vi "Settings Dialog.vi"(8 "error in (no error)":errorcluster, 9 "UI State":T1, 10 "Message Queues":T2, 11 "PRM State Cluster In":T6={"PRM Config"={"GUID"="", "Drop Coords"={"Horizontal"=0, "Vertical"=0}, "Process Name"="", "User name"="", "Queue Name"="", "Settings"={"Cycle Period"=500.0, "PID 2 Parameters"={"Input Device"=enum."Default", "Output Device"=enum."Default", "Setpoint"=0.0, "PID gains"={"proportional gain (Kc)"=1.0, "integral time (Ti, min)"=0.01, "derivative time (Td, min)"=0.0}, "output range"={"output low"=0.0, "output high"=100.0}}, "Manual Entry"=0.0, "Auto?"=TRUE, "4-20mA Input Settings"={"Input Channel "=0}, "4-20mA Out Settings"={"Output DAQ Task"=""}, "Input Channel Tag Name "=""}, "Settings Load Count"=0}, "State"=enum."Idle", "Start Time"=timestamp(0 s since 1904-01-01), "Current Time"=timestamp(0 s since 1904-01-01), "First Iteration"=FALSE, "Data"={"4-20mA Input"=0.0, "PID 2 Process Variable"=0.0, "PID 2 Output"=0.0, "4-20mA Output"=0.0}} {"PRM Config"."Settings"."PID 2 Parameters"."output range"."output low" format="%.2f"; "PRM Config"."Settings"."PID 2 Parameters"."output range"."output high" min=0.0 max=100.0 format="%.2f"; "PRM Config"."Settings"."PID 2 Parameters"."PID gains"."derivative time (Td, min)" format="%.3f"; "PRM Config"."Settings"."PID 2 Parameters"."PID gains"."integral time (Ti, min)" format="%.3f"; "PRM Config"."Settings"."PID 2 Parameters"."PID gains"."proportional gain (Kc)" format="%.3f"}) -> (0 "error out":errorcluster, 1 "Cancelled?":bool=TRUE, 2 "UI Refresh Needed?":bool, 3 "PRM State Cluster Out":T6={"PRM Config"={"GUID"="", "Drop Coords"={"Horizontal"=0, "Vertical"=0}, "Process Name"="", "User name"="", "Queue Name"="", "Settings"={"Cycle Period"=500.0, "PID 2 Parameters"={"Input Device"=enum."Default", "Output Device"=enum."Default", "Setpoint"=0.0, "PID gains"={"proportional gain (Kc)"=1.0, "integral time (Ti, min)"=0.01, "derivative time (Td, min)"=0.0}, "output range"={"output low"=0.0, "output high"=100.0}}, "Manual Entry"=0.0, "Auto?"=TRUE, "4-20mA Input Settings"={"Input Channel "=0}, "4-20mA Out Settings"={"Output DAQ Task"=""}, "Input Channel Tag Name "=""}, "Settings Load Count"=0}, "State"=enum."Idle", "Start Time"=timestamp(0 s since 1904-01-01), "Current Time"=timestamp(0 s since 1904-01-01), "First Iteration"=FALSE, "Data"={"4-20mA Input"=0.0, "PID 2 Process Variable"=0.0, "PID 2 Output"=0.0, "4-20mA Output"=0.0}} {"PRM Config"."Settings"."PID 2 Parameters"."output range"."output low" format="%.2f"; "PRM Config"."Settings"."PID 2 Parameters"."output range"."output high" min=0.0 max=100.0 format="%.2f"; "PRM Config"."Settings"."PID 2 Parameters"."PID gains"."derivative time (Td, min)" format="%.3f"; "PRM Config"."Settings"."PID 2 Parameters"."PID gains"."integral time (Ti, min)" format="%.3f"; "PRM Config"."Settings"."PID 2 Parameters"."PID gains"."proportional gain (Kc)" format="%.3f"})   [LabVIEW 2018, in "4-20mA Module.lvlib"]
uses:
  4-20mA Module.lvlib
  Controls/4-20mA Module State Cluster.ctl
  Controls/4-20mA Module Config Cluster.ctl
  <vilib>/Utility/miscctls.llb/LVPoint32TypeDef.ctl
  Controls/4-20mA Module Settings Cluster.ctl
  Pressure Transmitter/Pressure Transmitter Device Settings.ctl
  Pressure Reg Module/Pressure Regulator Device Settings.ctl
  Measure Instrument/State Enum.ctl
  Controls/4-20mA Message Queues.ctl
  support/Message Queue/Message Cluster.ctl
  controls/UI State.ctl
  Tag VIs/Tag FGV Operation Enum.ctl
  <vilib>/Utility/miscctls.llb/LVMinMaxIncTypeDef.ctl
  support/Message Queue/Enqueue Message (Single).vi
  Settings/Settings.lvlib
  Pressure Transmitter/Pressure Transmitter Library.lvlib
  Shared Variables/Dynamic Shared Variables.lvlib
  Pressure Reg Module/Pressure Regulator Library.lvlib
  support/Support Library.lvlib
  support/Message Queue/Message Queue.lvlib
  Flow Regulator/Pressure Reg Module/Flow Regulator Library.lvlib
  <vilib>/Utility/xml.llb/Write to XML File(string).vi
  Measure Instrument/Feed Module Engine.lvlib
panel:
  in  "Module Name":string
  in  "Start":bool
  in  "Stop":bool
  in  "Pressure Regulator Configuration":T5={"Cycle Period"=500.0, "PID 2 Parameters"={"Input Device"=enum."Default", "Output Device"=enum."Default", "Setpoint PSIA"=0.0, "PID gains"={"proportional gain (Kc)"=1.0, "integral time (Ti, min)"=0.01, "derivative time (Td, min)"=0.0}, "output range"={"output low"=0.0, "output high"=100.0}}, "Manual PSIA"=0.0, "Auto?"=TRUE, "4-20mA Input Settings"={"Input Channel "=0}, "Out Settings"={"Output DAQ Task"=""}, "Simulated"=FALSE} {"4-20mA Input Settings"."Input Channel" items=["Default", "TT0", "PT0", "PR 1:4-20mA Input", "PR 1:PID2Out", "PR 1:4-20mA Output", "PR 1:Input Device Disconnected", "PR 1:Output Device Disconnected"]; "Manual PSIA" min=0.0 max=50.0; "PID 2 Parameters"."output range"."output low" format="%.2f"; "PID 2 Parameters"."output range"."output high" min=0.0 max=100.0 format="%.2f"; "PID 2 Parameters"."PID gains"."derivative time (Td, min)" format="%.3f"; "PID 2 Parameters"."PID gains"."integral time (Ti, min)" format="%.3f"; "PID 2 Parameters"."PID gains"."proportional gain (Kc)" format="%.3f"}
  in  "Cancel Button":bool
  in  "OK Button":bool
  # "Output Settings"
  # "Input Settings"
  # "Instrument Settings"
  # "Instrument Settings"
  # "Instrument Settings"
  # "Instrument Settings"
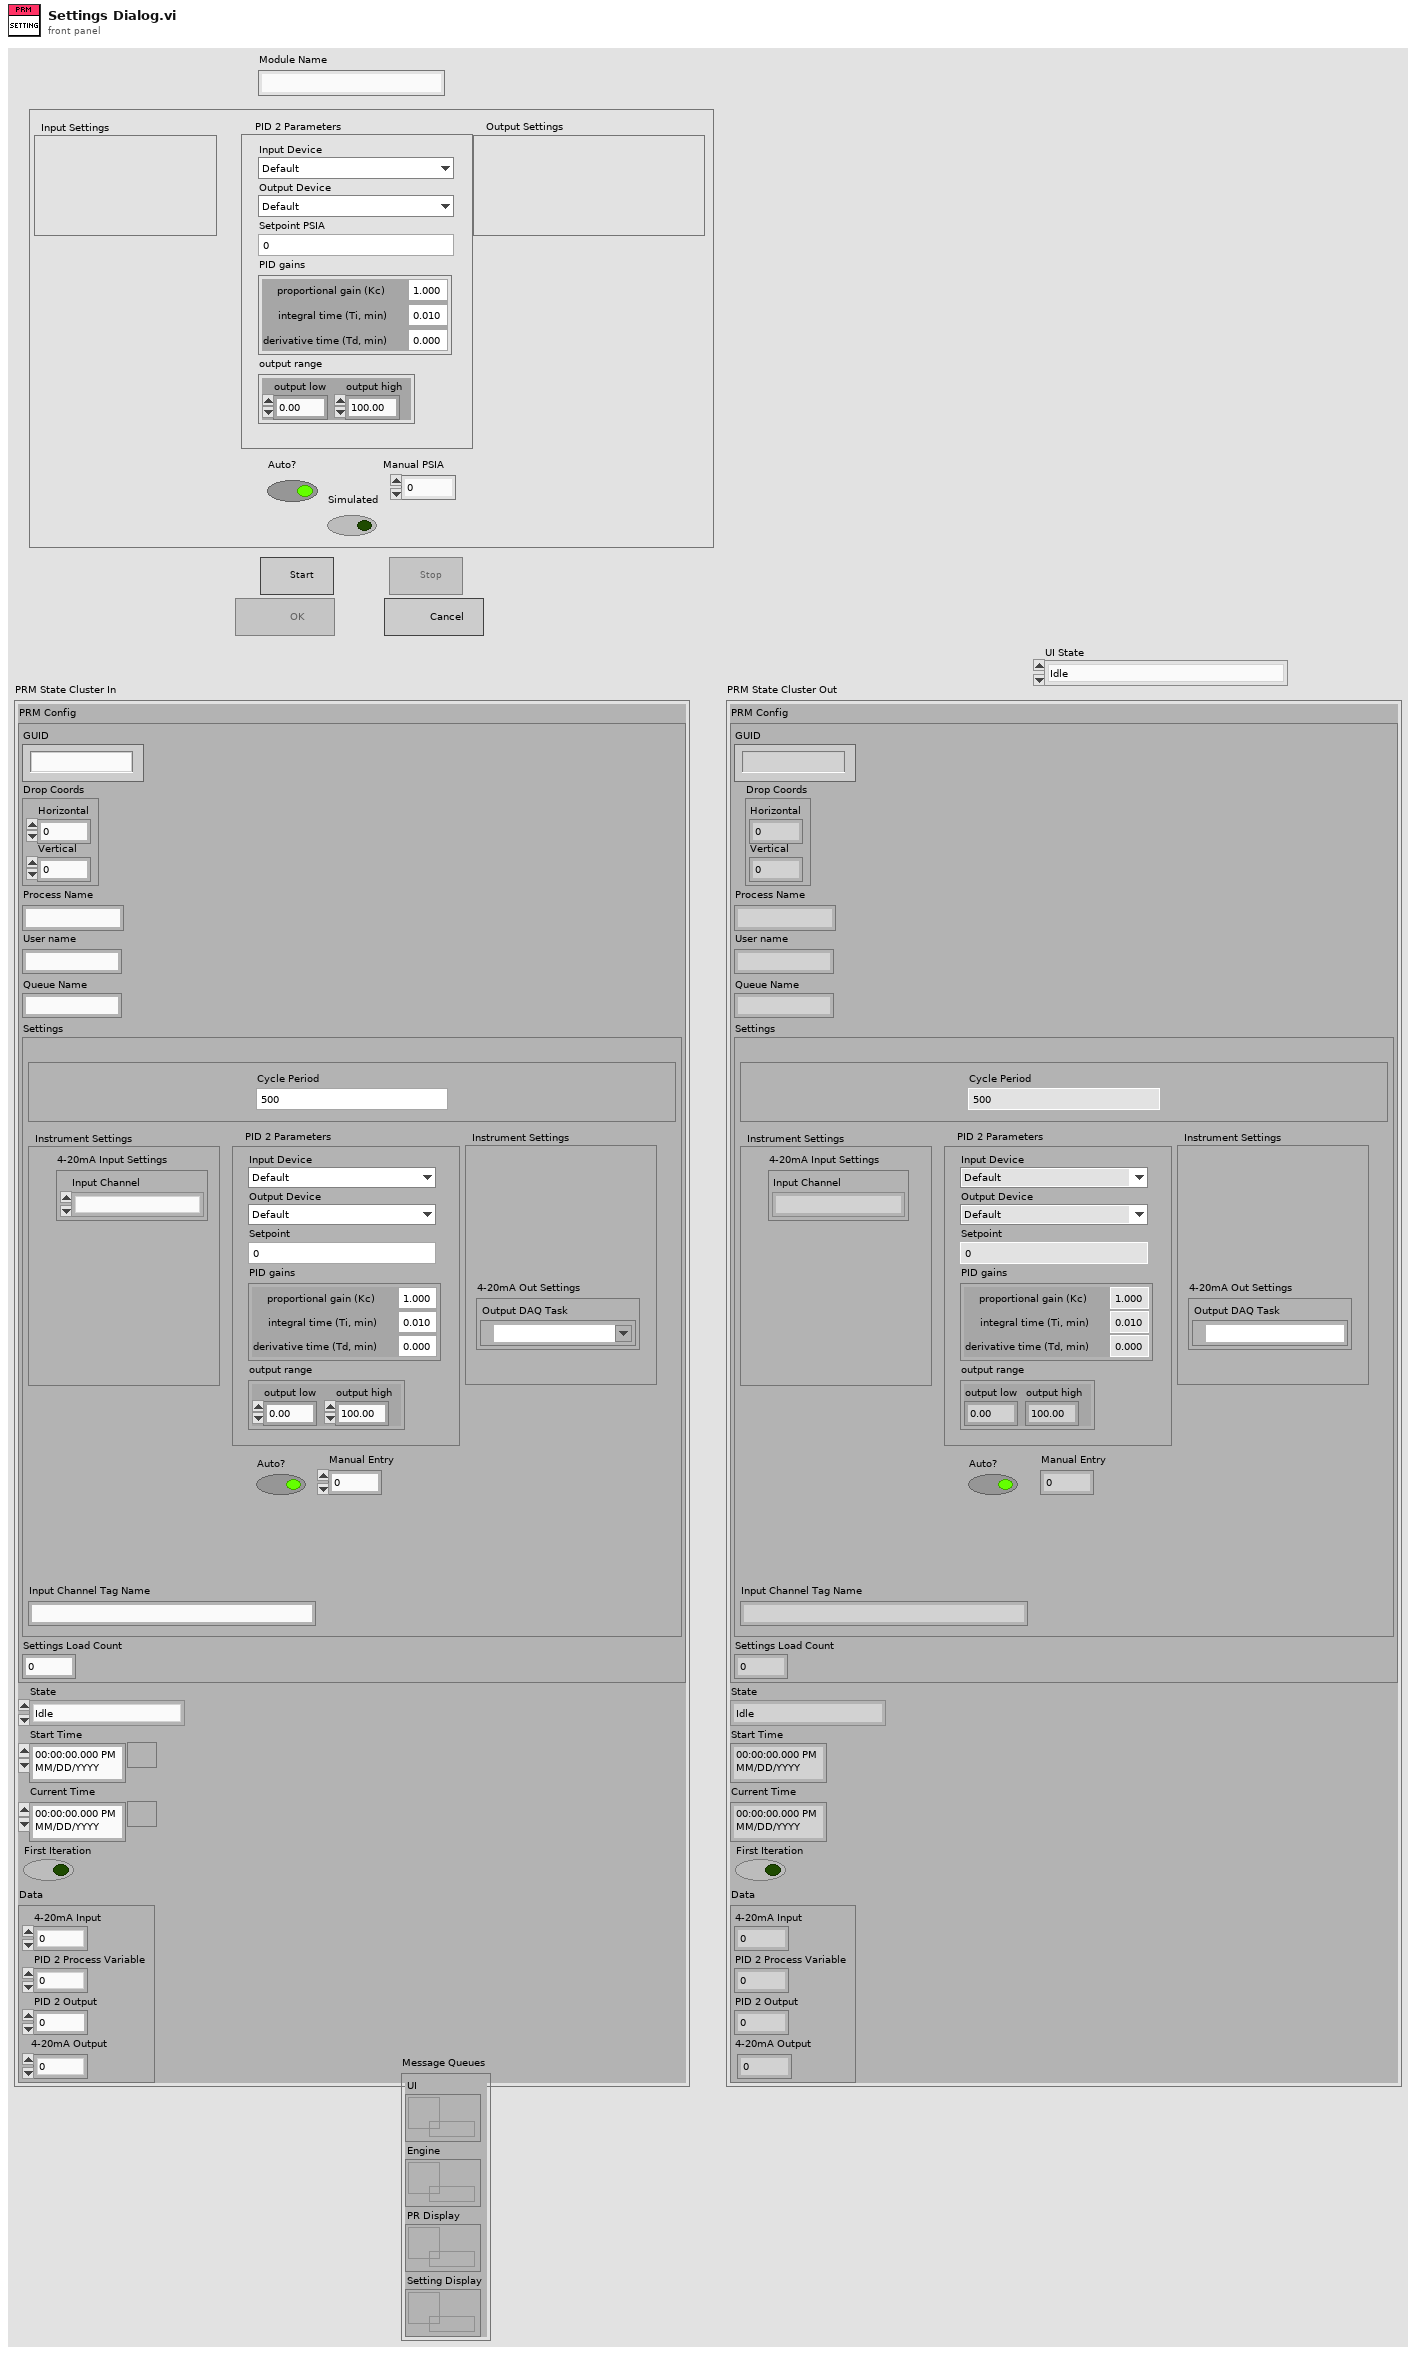
[diagram p1: front panel]
types:
  T1 = typedef "UI State.ctl" = enum16{"Idle", "Acquiring and Logging", "Waiting for Exit", "Waiting for Exit (Acq Stopped)", "Waiting for Exit (Log Stopped)", "Waiting for Stop", "Waiting for Stop (Acq Stopped)", "Waiting for Stop (Log Stopped)"}
  T2 = typedef "4-20mA Module.lvlib/4-20mA Message Queues.ctl" = cluster{"UI":refnum<queue>, "Engine":refnum<queue>, "PR Display":refnum<queue>, "Setting Display":refnum<queue>}
  T3 = typedef "Pressure Transmitter Library.lvlib/Pressure Transmitter Device Settings.ctl" = cluster{"Input Channel ":u16}
  T4 = typedef "Pressure Regulator Library.lvlib/Pressure Regulator Device Settings.ctl" = cluster{"Output DAQ Task":refnum<k21>}
  T5 = cluster{"Cycle Period":dbl, "PID 2 Parameters":cluster{"Input Device":enum16{"Default", "4-20mA"}, "Output Device":enum16{"Default", "Equilibar Pressure Reg", "Flow Regulator"}, "Setpoint PSIA":dbl, "PID gains":cluster{"proportional gain (Kc)":dbl, "integral time (Ti, min)":dbl, "derivative time (Td, min)":dbl}, "output range":cluster{"output low":dbl, "output high":dbl}}, "Manual PSIA":dbl, "Auto?":bool, "4-20mA Input Settings":T3, "Out Settings":T4, "Simulated":bool}
  T6 = typedef "4-20mA Module.lvlib/4-20mA Module State Cluster.ctl" = cluster{"PRM Config":T7, "State":T10, "Start Time":timestamp, "Current Time":timestamp, "First Iteration":bool, "Data":cluster{"4-20mA Input":dbl, "PID 2 Process Variable":dbl, "PID 2 Output":dbl, "4-20mA Output":dbl}}
  T7 = typedef "4-20mA Module.lvlib/4-20mA Module Config Cluster.ctl" = cluster{"GUID":string, "Drop Coords":T8, "Process Name":string, "User name":string, "Queue Name":string, "Settings":T9, "Settings Load Count":i32}
  T8 = typedef "LVPoint32TypeDef.ctl" = cluster{"Horizontal":i32, "Vertical":i32}
  T9 = typedef "4-20mA Module.lvlib/4-20mA Module Settings Cluster.ctl" = cluster{"Cycle Period":dbl, "PID 2 Parameters":cluster{"Input Device":enum16{"Default", "4-20mA"}, "Output Device":enum16{"Default", "Equilibar Pressure Reg", "Flow Regulator"}, "Setpoint":dbl, "PID gains":cluster{"proportional gain (Kc)":dbl, "integral time (Ti, min)":dbl, "derivative time (Td, min)":dbl}, "output range":cluster{"output low":dbl, "output high":dbl}}, "Manual Entry":dbl, "Auto?":bool, "4-20mA Input Settings":T3, "4-20mA Out Settings":T4, "Input Channel Tag Name ":string}
  T10 = typedef "Feed Module.lvlib/Feed Module Engine.lvlib/State Enum.ctl" = enum16{"Measuring", "Idle", "Paused"}
  T11 = typedef "Tag FGV Operation Enum.ctl" = enum16{"Init", "Set Notification Queue", "Create Tag", "Commit", "Write Tag (Numeric)", "Write Tag (Boolean)", "Read All Tags", "Read One Tag", "Delete Tag Category", "Set Alarm Parameters (Numeric)", "Set Alarm Parameters (Boolean)", "Enable All Alarms", "Disable All Alarms", "Delete All Tags", "Read Alarms", "Ack Alarm", "Read Alarm Parameters (Numeric)", "Read Alarm Parameters (Boolean)"}
  T12 = enum8{"Enabled", "Disabled", "Disabled and Grayed Out"}
  T13 = typedef "LVMinMaxIncTypeDef.ctl" = cluster{"Minimum":dbl, "Maximum":dbl, "Increment":dbl}
  T14 = cluster{"Input Device":enum16{"Default", "4-20mA"}, "Output Device":enum16{"Default", "Equilibar Pressure Reg", "Flow Regulator"}, "Setpoint":dbl, "PID gains":cluster{"proportional gain (Kc)":dbl, "integral time (Ti, min)":dbl, "derivative time (Td, min)":dbl}, "output range":cluster{"output low":dbl, "output high":dbl}}
  T15 = cluster{"Input Device":enum16{"Default", "4-20mA"}, "Output Device":enum16{"Default", "Equilibar Pressure Reg", "Flow Regulator"}, "Setpoint PSIA":dbl, "PID gains":cluster{"proportional gain (Kc)":dbl, "integral time (Ti, min)":dbl, "derivative time (Td, min)":dbl}, "output range":cluster{"output low":dbl, "output high":dbl}}
  T16 = enum16{"Default", "Equilibar Pressure Reg", "Flow Regulator"}
  T17 = cluster{"Numeric Text.Text":dbl, "Numeric Text.Text":dbl, "Numeric Text.Text":dbl}
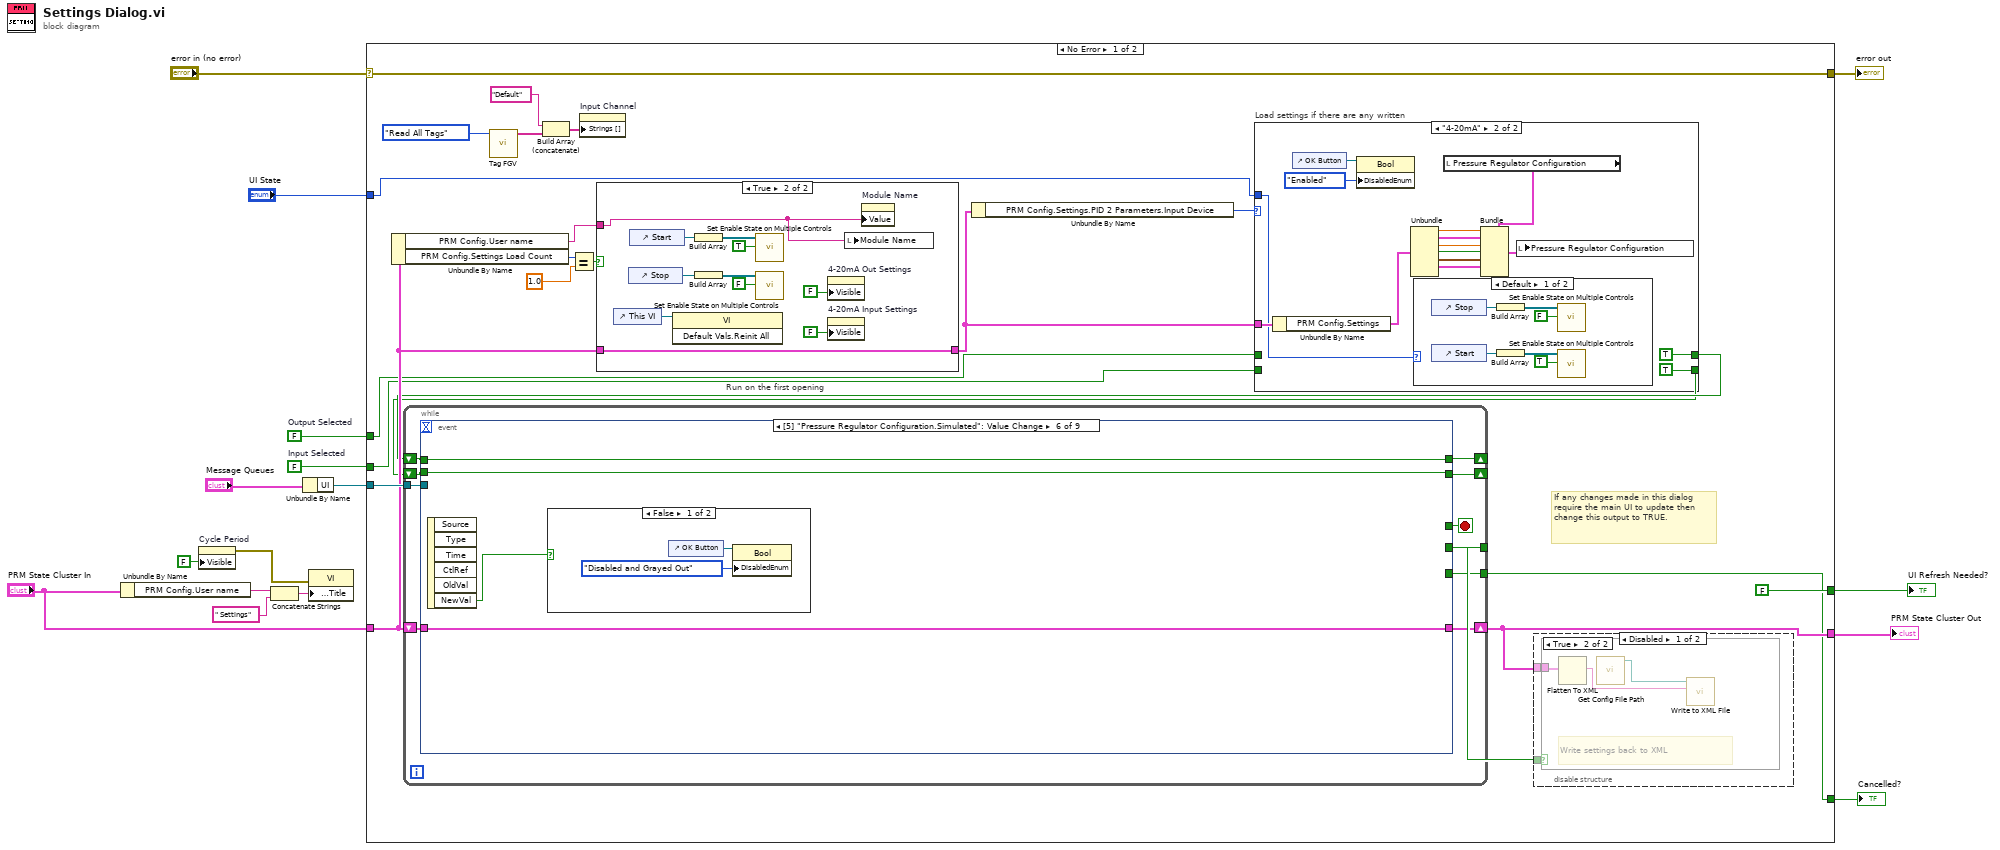
[diagram p0: block diagram]
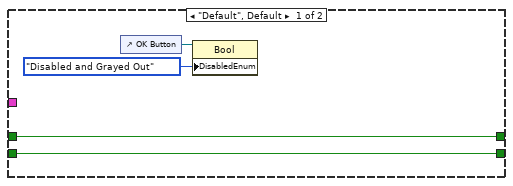
[diagram p4: hidden frame]
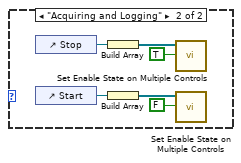
[diagram p5: hidden frame]
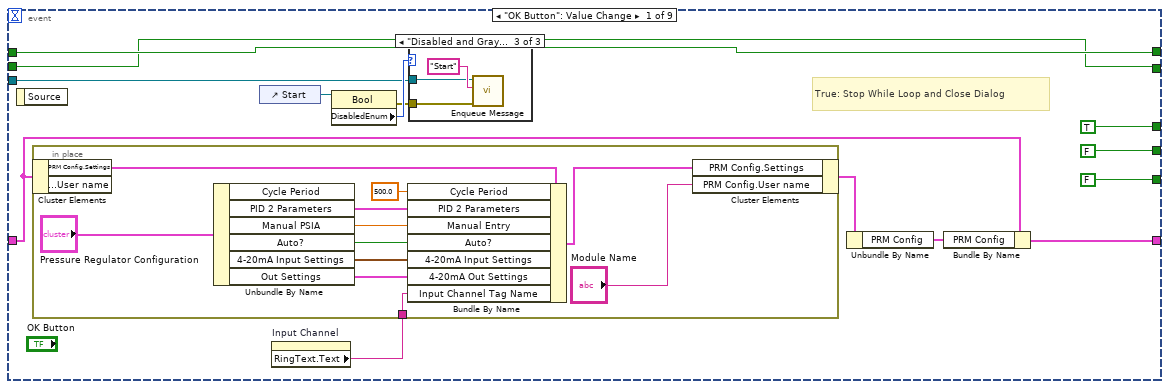
[diagram p7: hidden frame]
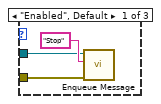
[diagram p8: hidden frame]
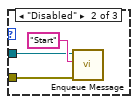
[diagram p9: hidden frame]
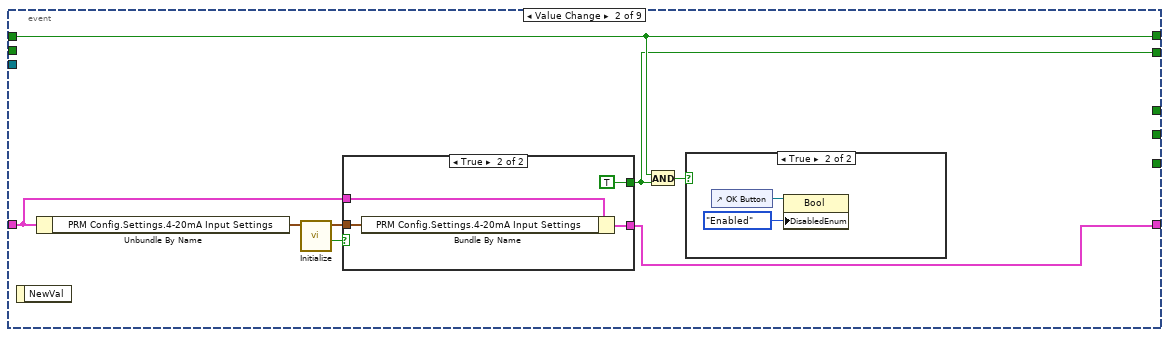
[diagram p10: hidden frame]
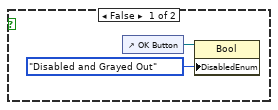
[diagram p11: hidden frame]
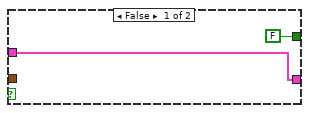
[diagram p12: hidden frame]
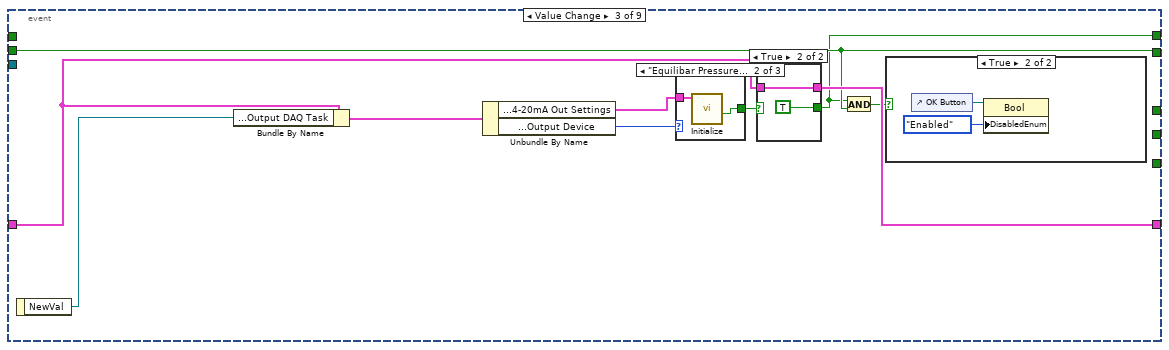
[diagram p13: hidden frame]
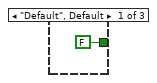
[diagram p14: hidden frame]
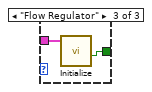
[diagram p15: hidden frame]
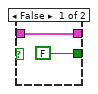
[diagram p16: hidden frame]
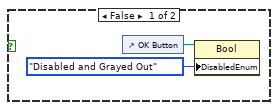
[diagram p17: hidden frame]
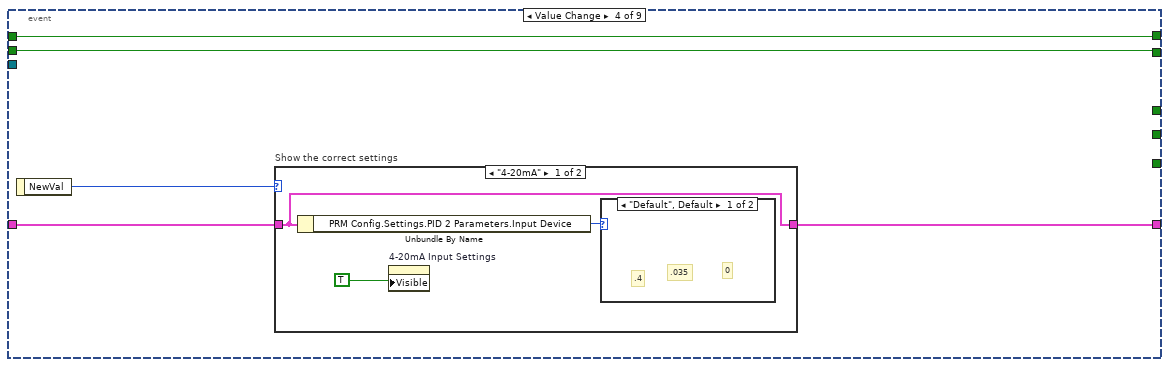
[diagram p18: hidden frame]
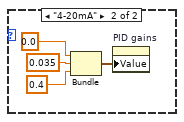
[diagram p19: hidden frame]
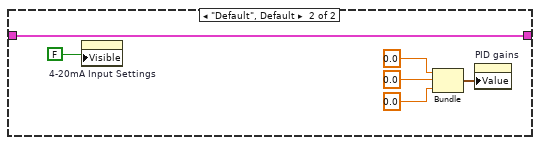
[diagram p20: hidden frame]
diagram:
  w5 = FALSE  # Input Selected
  w6 = FALSE  # Output Selected
  n1 = Unbundle By Name("PRM State Cluster In") -> ("PRM Config.User name"=w13:string)
  n2 = property on="Cycle Period" class="DigNum (strict)"("Visible"=FALSE) -> (error out=w1:errorcluster)  [unwired: 2 in, 1 out]
  n3 = Concatenate Strings(w13, " Settings" ("string")) -> (w12:string)
  n4 = Unbundle By Name("Message Queues") -> ("UI"=w7:refnum<queue>)
  n5 = property class="VI"(error in=w1, "Front Panel.Title"=w12) -> ()  [unwired: 1 in, 2 out]
  n6 = case shown="No Error" "error in (no error)" {
    selector: "error in (no error)" -> [w38 w237]
    tunnel: [w38 w237] -> w16
    tunnel: "PRM State Cluster In" -> [w25 w236]
    tunnel: [w36 w236] -> w10
    tunnel: [FALSE ("UI Refresh Needed?") _] -> w15
    tunnel: [w35 TRUE ("UI Refresh Needed?")] -> w14
    tunnel: w7 -> [w26 _]
    tunnel: w6 -> [w24 _]
    tunnel: w5 -> [w23 _]
    tunnel: "UI State" -> [w20 _]
    frame No Error {
      # "If any changes made in this dialog require the main UI to update then change this output to TRUE."
      n7 = Unbundle By Name(w25) -> ("PRM Config.User name"=w19:string, "PRM Config.Settings Load Count"=w34:i32)
      n8 = call "Tag FGV.vi"("Operation"=Tag_FGV_Operation_Enum."Read All Tags") -> ("Tag Names"=w18:string[])  [unwired: 7 in, 7 out]
      n9 = Build Array (concatenate)("Default", w18) -> (w27:string[])
      n10 = Equal?(x=w34, y=1.0) -> (x = y?=w31:bool)
      n11 = property on="Input Channel" class="Ring (strict)"("Strings []"=w27) -> ()  [unwired: 2 in, 2 out]
      n12 = case "Run on the first opening" shown="True" w31 {
        tunnel: w25 -> [w75 w85]
        tunnel: [w75 w85] -> w29
        tunnel: w19 -> [_ w76]
        frame False {
        }
        frame True {
          n13 = control-ref of="This VI"() -> (w86:refnum<vi>)
          n14 = control-ref of="Stop"() -> (w81:refnum<vi>)
          n15 = control-ref of="Start"() -> (w82:refnum<vi>)
          n16 = invoke class="VI" method="Default Vals.Reinit All"(reference=w86) -> ()  [unwired: 2 in, 3 out]
          n17 = Build Array(w82) -> (w80:refnum<vi>[])
          n18 = Build Array(w81) -> (w79:refnum<vi>[])
          n19 = call "Set Enable State on Multiple Controls.vi"("Enable?"=TRUE, "Controls"=w80) -> ()  [unwired: 10 in]
          n20 = call "Set Enable State on Multiple Controls.vi"("Enable?"=FALSE, "Controls"=w79) -> ()  [unwired: 10 in]
          n21 = property on="4-20mA Out Settings" class="Clust (strict)"("Visible"=FALSE) -> ()  [unwired: 2 in, 2 out]
          n22 = property on="4-20mA Input Settings" class="Clust (strict)"("Visible"=FALSE) -> ()  [unwired: 2 in, 2 out]
          n23 = local write "Module Name"(w76) -> ()
          n24 = property on="Module Name" class="Str"("Value"=w76) -> ()  [unwired: 2 in, 2 out]
        }
      }
      n25 = Unbundle By Name(w29) -> ("PRM Config.Settings.PID 2 Parameters.Input Device"=w30:enum16{"Default", "4-20mA"})
      n26 = case "Load settings if there are any written" shown="\"4-20mA\"" w30 {
        tunnel: w29 -> [_ w56]
        tunnel: w24 -> [w45 _]
        tunnel: w23 -> [w44 _]
        tunnel: [w45 TRUE] -> w22
        tunnel: [w44 TRUE] -> w21
        tunnel: w20 -> [_ w49]
        frame "Default", Default {
          n27 = control-ref of="OK Button"() -> (w47:refnum<vi>)
          n28 = property on="Property Node" class="Bool"(reference=w47, "DisabledEnum"=T12."Disabled and Grayed Out" ("Disabled")) -> ()  [unwired: 1 in, 2 out]
        }
        frame "4-20mA" {
          n29 = Unbundle By Name(w56) -> ("PRM Config.Settings"=w60:T9)
          n30 = control-ref of="OK Button"() -> (w54:refnum<vi>)
          n31 = property on="Property Node" class="Bool"(reference=w54, "DisabledEnum"=T12."Enabled" ("Disabled")) -> ()  [unwired: 1 in, 2 out]
          n32 = Unbundle(w60) -> ("Cycle Period"=w61:dbl, "PID 2 Parameters"=w62:T14, "Manual Entry"=w57:dbl, "Auto?"=w58:bool, "4-20mA Input Settings"=w59:T3, "4-20mA Out Settings"=w52:T4)  [unwired: 1 out]
          n33 = case shown="Default" w49 {
            frame Default {
              n34 = control-ref of="Stop"() -> (w66:refnum<vi>)
              n35 = control-ref of="Start"() -> (w67:refnum<vi>)
              n36 = Build Array(w66) -> (w65:refnum<vi>[])
              n37 = Build Array(w67) -> (w68:refnum<vi>[])
              n38 = call "Set Enable State on Multiple Controls.vi"("Enable?"=FALSE, "Controls"=w65) -> ()  [unwired: 10 in]
              n39 = call "Set Enable State on Multiple Controls.vi"("Enable?"=TRUE, "Controls"=w68) -> ()  [unwired: 10 in]
            }
            frame "Acquiring and Logging" {
              n40 = control-ref of="Stop"() -> (w72:refnum<vi>)
              n41 = control-ref of="Start"() -> (w73:refnum<vi>)
              n42 = Build Array(w72) -> (w71:refnum<vi>[])
              n43 = Build Array(w73) -> (w74:refnum<vi>[])
              n44 = call "Set Enable State on Multiple Controls.vi"("Enable?"=TRUE, "Controls"=w71) -> ()  [unwired: 10 in]
              n45 = call "Set Enable State on Multiple Controls.vi"("Enable?"=FALSE, "Controls"=w74) -> ()  [unwired: 10 in]
            }
          }
          n46 = local read "Pressure Regulator Configuration"() -> (w48:T5)
          n47 = Bundle(cluster=w48, "Cycle Period"=w61, "PID 2 Parameters"=w62, "Manual PSIA"=w57, "Auto?"=w58, "4-20mA Input Settings"=w59, "Out Settings"=w52) -> (w55:T5)  [unwired: 1 in]
          n48 = local write "Pressure Regulator Configuration"(w55) -> ()
        }
      }
      n49 = while {
        tunnel: [w96] -> w32
        tunnel: [w93] -> w35
        tunnel: w26 -> [w92]
        shift-right: [w88] -> _
        shift-left: w22 -> [w91]
        shift-right: [w89] -> _
        shift-left: w21 -> [w90]
        shift-right: [w95] -> w36
        shift-left: w25 -> [w87]
        stop <- w94 stop-if-true
        n50 = event shown="[5] \"Pressure Regulator Configuration.Simulated\": Value Change" {
          selector: _ -> [_ _ _ _ _ _ _ _ _]
          dyn-events: _ -> [_ _ _ _ _ _ _ _ _]
          timeout: _ -> [_ _ _ _ _ _ _ _ _]
          tunnel: [w106 w138 w158 w176 w190 w203 w208 w225 w234] -> w95
          tunnel: w87 -> [w98 w135 w152 w175 w192 w203 w209 w225 w234]
          tunnel: [FALSE ("UI Refresh Needed?") _ _ _ _ _ FALSE ("UI Refresh Needed?") _ _] -> w96
          tunnel: [TRUE _ _ _ _ _ TRUE _ _] -> w94
          tunnel: [FALSE ("UI Refresh Needed?") _ _ _ _ _ TRUE ("UI Refresh Needed?") _ _] -> w93
          tunnel: w92 -> [w102 _ _ _ _ _ _ _ _]
          tunnel: w91 -> [w100 w132 _ w173 w194 w201 w211 w218 w227]
          tunnel: w90 -> [w99 _ w154 w172 w193 w202 w210 w217 w226]
          tunnel: [w99 w131 w154 w172 w193 w202 w210 w217 w226] -> w89
          tunnel: [w100 w132 w150 w173 w194 w201 w211 w218 w227] -> w88
          event "OK Button": Value Change {
            # "True: Stop While Loop and Close Dialog"
            n51 = event-data() -> ()  [unwired: 1 in, 1 out]
            n52 = control-ref of="Start"() -> (w101:refnum<vi>)
            n53 = property on="Input Channel" class="Ring (strict)"() -> ("RingText.Text"=w105:string)  [unwired: 2 in, 2 out]
            n54 = in-place {
              in-place-border: w105 -> [w115]
              n55 = in-place-cluster #1(w98) -> ("PRM Config.Settings"=w111:T9)  [unwired: 1 out]
              n56 = Unbundle By Name("Pressure Regulator Configuration") -> ("PID 2 Parameters"=w120:T15, "Manual PSIA"=w119:dbl, "Auto?"=w118:bool, "4-20mA Input Settings"=w117:T3, "Out Settings"=w116:T4)  [unwired: 1 out]
              n57 = Bundle By Name(cluster=w111, "Cycle Period"=500.0, "PID 2 Parameters"=w120, "Manual Entry"=w119, "Auto?"=w118, "4-20mA Input Settings"=w117, "4-20mA Out Settings"=w116, "Input Channel Tag Name"=w115) -> (w112:T9)
              n58 = in-place-cluster #1("PRM Config.Settings"=w112, "PRM Config.User name"="Module Name") -> (w97:T6)
            }
            n59 = property class="Bool"(reference=w101) -> (error out=w103:errorcluster, "DisabledEnum"=w104:T12)  [unwired: 1 in, 1 out]
            n60 = case shown="\"Disabled and Grayed Out\"" w104 {
              tunnel: w103 -> [w123 w126 w129]
              tunnel: w102 -> [w122 w125 w128]
              frame "Enabled", Default {
                n61 = call-poly "Enqueue Message.vi"("error in (no error)"=w123, "Message"="Stop", "Message Queue"=w122) -> ()  [unwired: 7 in, 2 out]
              }
              frame "Disabled" {
                n62 = call-poly "Enqueue Message.vi"("error in (no error)"=w126, "Message"="Start", "Message Queue"=w125) -> ()  [unwired: 7 in, 2 out]
              }
              frame "Disabled and Grayed Out" {
                n63 = call-poly "Enqueue Message.vi"("error in (no error)"=w129, "Message"="Start", "Message Queue"=w128) -> ()  [unwired: 7 in, 2 out]
              }
            }
            n64 = Unbundle By Name(w97) -> ("PRM Config"=w107:T7)
            n65 = Bundle By Name(cluster=w98, "PRM Config"=w107) -> (w106:T6)
          }
          event Value Change {
            n66 = event-data() -> ()  [unwired: 1 in, 1 out]
            n67 = Unbundle By Name(w135) -> ("PRM Config.Settings.4-20mA Input Settings"=w134:T3)
            n68 = call "Initialize.vi"("4-20mA Settings In"=w134) -> ("Initialized"=w137:bool, "4-20mA Settings Out"=w136:T3)  [unwired: 8 in, 1 out]
            n69 = case shown="True" w137 {
              tunnel: w135 -> [w144 w148]
              tunnel: [w144 w146] -> w138
              tunnel: w136 -> [_ w147]
              tunnel: [FALSE TRUE] -> w131
              frame False {
              }
              frame True {
                n70 = Bundle By Name(cluster=w148, "PRM Config.Settings.4-20mA Input Settings"=w147) -> (w146:T6)
              }
            }
            n71 = And(x=w132, y=w131) -> (x .and. y?=w133:bool)
            n72 = case shown="True" w133 {
              frame False {
                n73 = control-ref of="OK Button"() -> (w140:refnum<vi>)
                n74 = property on="Property Node" class="Bool"(reference=w140, "DisabledEnum"=T12."Disabled and Grayed Out" ("Disabled")) -> ()  [unwired: 1 in, 2 out]
              }
              frame True {
                n75 = control-ref of="OK Button"() -> (w142:refnum<vi>)
                n76 = property on="Property Node" class="Bool"(reference=w142, "DisabledEnum"=T12."Enabled" ("Disabled")) -> ()  [unwired: 1 in, 2 out]
              }
            }
          }
          event Value Change {
            n77 = event-data() -> ("NewVal"=w153:refnum<k21>)  [unwired: 1 in]
            n78 = Bundle By Name(cluster=w152, "PRM Config.Settings.4-20mA Out Settings.Output DAQ Task"=w153) -> (w151:T6)
            n79 = Unbundle By Name(w151) -> ("PRM Config.Settings.4-20mA Out Settings"=w157:T4, "PRM Config.Settings.PID 2 Parameters.Output Device"=w149:T16)
            n80 = case shown="\"Equilibar Pressure Reg\"" w149 {
              tunnel: w157 -> [_ w161 w163]
              tunnel: [FALSE ("Initialized") w160 w162] -> w155
              frame "Default", Default {
              }
              frame "Equilibar Pressure Reg" {
                n81 = call "Initialize.vi"("4-20mA Out Settings In"=w161) -> ("Initialized"=w160:bool)  [unwired: 8 in, 2 out]
              }
              frame "Flow Regulator" {
                n82 = call "Initialize.vi"("4-20mA Out Settings In"=w163) -> ("Initialized"=w162:bool)  [unwired: 8 in, 2 out]
              }
            }
            n83 = case shown="True" w155 {
              tunnel: [w165 w166] -> w158
              tunnel: w152 -> [w165 w166]
              tunnel: [FALSE TRUE] -> w150
              frame False {
              }
              frame True {
              }
            }
            n84 = And(x=w150, y=w154) -> (x .and. y?=w156:bool)
            n85 = case shown="True" w156 {
              frame False {
                n86 = control-ref of="OK Button"() -> (w168:refnum<vi>)
                n87 = property on="Property Node" class="Bool"(reference=w168, "DisabledEnum"=T12."Disabled and Grayed Out" ("Disabled")) -> ()  [unwired: 1 in, 2 out]
              }
              frame True {
                n88 = control-ref of="OK Button"() -> (w170:refnum<vi>)
                n89 = property on="Property Node" class="Bool"(reference=w170, "DisabledEnum"=T12."Enabled" ("Disabled")) -> ()  [unwired: 1 in, 2 out]
              }
            }
          }
          event "Pressure Regulator Configuration.PID 2 Parameters.Input Device": Value Change {
            n90 = event-data() -> ("NewVal"=w174:enum16{"Default", "4-20mA"})  [unwired: 1 in]
            n91 = case "Show the correct settings" shown="\"4-20mA\"" w174 {
              tunnel: [w178 w189] -> w176
              tunnel: w175 -> [w178 w189]
              frame "4-20mA" {
                n92 = Unbundle By Name(w178) -> ("PRM Config.Settings.PID 2 Parameters.Input Device"=w179:enum16{"Default", "4-20mA"})
                n93 = property on="4-20mA Input Settings" class="Clust (strict)"("Visible"=TRUE) -> ()  [unwired: 2 in, 2 out]
                n94 = case shown="\"Default\", Default" w179 {
                  frame "Default", Default {
                    # "0"
                    # ".035"
                    # ".4"
                  }
                  frame "4-20mA" {
                    n95 = Bundle("Numeric Text.Text"=0.0, "Numeric Text.Text"=0.035, "Numeric Text.Text"=0.4) -> (w180:T17)  [unwired: 1 in]
                    n96 = property on="PID gains" class="Clust (strict)"("Value"=w180) -> ()  [unwired: 2 in, 2 out]
                  }
                }
              }
              frame "Default", Default {
                n97 = property on="4-20mA Input Settings" class="Clust (strict)"("Visible"=FALSE) -> ()  [unwired: 2 in, 2 out]
                n98 = Bundle("Numeric Text.Text"=0.0, "Numeric Text.Text"=0.0, "Numeric Text.Text"=0.0) -> (w187:T17)  [unwired: 1 in]
                n99 = property on="PID gains" class="Clust (strict)"("Value"=w187) -> ()  [unwired: 2 in, 2 out]
              }
            }
          }
          event "Pressure Regulator Configuration.PID 2 Parameters.Output Device": Value Change {
            n100 = event-data() -> ("NewVal"=w191:T16)  [unwired: 1 in]
            n101 = Bundle By Name(cluster=w192, "PRM Config.Settings.PID 2 Parameters.Output Device"=w191) -> (w190:T6)
            n102 = case "Show the correct settings" shown="\"Equilibar Pressure Reg\"" w191 {
              frame "Equilibar Pressure Reg" {
                n103 = property on="4-20mA Out Settings" class="Clust (strict)"("Visible"=TRUE) -> ()  [unwired: 2 in, 2 out]
                n104 = property on="Manual PSIA" class="DigNum (strict)"("Data Range"=T13 {"Minimum"=0.0, "Maximum"=50.0, "Increment"=0.0} ("Data Entry Limits")) -> ()  [unwired: 2 in, 2 out]
              }
              frame "Flow Regulator" {
                n105 = property on="4-20mA Out Settings" class="Clust (strict)"("Visible"=TRUE) -> ()  [unwired: 2 in, 2 out]
                n106 = property on="Manual PSIA" class="DigNum (strict)"("Data Range"=T13 {"Minimum"=0.0, "Maximum"=1000.0, "Increment"=0.0} ("Data Entry Limits")) -> ()  [unwired: 2 in, 2 out]
              }
              frame "Default", Default {
                n107 = property on="4-20mA Out Settings" class="Clust (strict)"("Visible"=FALSE) -> ()  [unwired: 2 in, 2 out]
              }
            }
          }
          event "Pressure Regulator Configuration.Simulated": Value Change {
            n108 = event-data() -> ("NewVal"=w200:bool)  [unwired: 1 in, 5 out]
            n109 = case shown="False" w200 {
              frame False {
                n110 = control-ref of="OK Button"() -> (w205:refnum<vi>)
                n111 = property on="Property Node" class="Bool"(reference=w205, "DisabledEnum"=T12."Disabled and Grayed Out" ("Disabled")) -> ()  [unwired: 1 in, 2 out]
              }
              frame True {
                n112 = control-ref of="OK Button"() -> (w207:refnum<vi>)
                n113 = property on="Property Node" class="Bool"(reference=w207, "DisabledEnum"=T12."Enabled" ("Disabled")) -> ()  [unwired: 1 in, 2 out]
              }
            }
          }
          event "Cancel Button": Value Change; Panel Close {
            # "True: Stop While Loop and Close Dialog"
            n114 = event-data() -> ()  [unwired: 1 in, 1 out]
            n115 = in-place {
              n116 = in-place-cluster #2(w209) -> ("PRM Config.Settings Load Count"=w215:i32)
              n117 = Decrement(x=w215) -> (x-1=w216:i32)
              n118 = in-place-cluster #2("PRM Config.Settings Load Count"=w216) -> (w208:T6)
            }
          }
          event "Start": Value Change {
            n119 = event-data() -> ()  [unwired: 1 in, 4 out]
            n120 = control-ref of="Start"() -> (w220:refnum<vi>)
            n121 = control-ref of="Stop"() -> (w219:refnum<vi>)
            n122 = Build Array(w220) -> (w221:refnum<vi>[])
            n123 = Build Array(w219) -> (w224:refnum<vi>[])
            n124 = call "Set Enable State on Multiple Controls.vi"("Enable?"=FALSE, "Controls"=w221) -> ()  [unwired: 10 in]
            n125 = call "Set Enable State on Multiple Controls.vi"("Enable?"=TRUE, "Controls"=w224) -> ()  [unwired: 10 in]
          }
          event "Stop": Value Change {
            n126 = event-data() -> ()  [unwired: 1 in, 4 out]
            n127 = control-ref of="Stop"() -> (w231:refnum<vi>)
            n128 = control-ref of="Start"() -> (w230:refnum<vi>)
            n129 = Build Array(w231) -> (w233:refnum<vi>[])
            n130 = Build Array(w230) -> (w229:refnum<vi>[])
            n131 = call "Set Enable State on Multiple Controls.vi"("Enable?"=FALSE, "Controls"=w233) -> ()  [unwired: 10 in]
            n132 = call "Set Enable State on Multiple Controls.vi"("Enable?"=TRUE, "Controls"=w229) -> ()  [unwired: 10 in]
          }
        }
      }
      n133 = disable-structure shown="Disabled" {
        disable-tunnel: w36 -> [w40 _]
        disable-tunnel: w32 -> [w39 _]
        frame Disabled {
          n134 = case shown="True" w39 {
            tunnel: w40 -> [_ w42]
            frame False {
            }
            frame True {
              # "Write settings back to XML"
              n135 = Flatten To XML(anything=w42) -> (xml string=w41:string)
              n136 = call "Get Config File Path.vi"() -> ("XML File Path"=w43:path)  [unwired: 10 in, 1 out]
              n137 = call-poly <vilib>:"Write to XML File.vi"("XML Input"=w41, "XML File Path"=w43) -> ()  [unwired: 7 in, 3 out]
            }
          }
        }
        frame Enabled {
        }
      }
    }
    frame Error {
    }
  }
  "UI Refresh Needed?" <- w15
  "error out" <- w16
  "Cancelled?" <- w14
  "PRM State Cluster Out" <- w10
